vi "Simple Reader.vi"(8 "error in (no error)":errorcluster, 11 "ITC-503 Driver in":refnum<class "ITC-503 Driver.lvclass">) -> (0 "error out":errorcluster, 2 "Signals":dbl[](array[numeric]), 3 "ITC-503 Driver out":refnum<class "ITC-503 Driver.lvclass">)   [LabVIEW 2025, in "ITC-503 Driver.lvclass"]
uses:
  ITC-503 Driver.lvclass
  VISA Instrument/VISA Instrument.lvclass/VISA Instrument.ctl
  VISA Instrument/Read VISA resource.vi
  VISA Instrument/Write VISA resource.vi
  Temperature Controller Driver/Read T controller configuration.vi
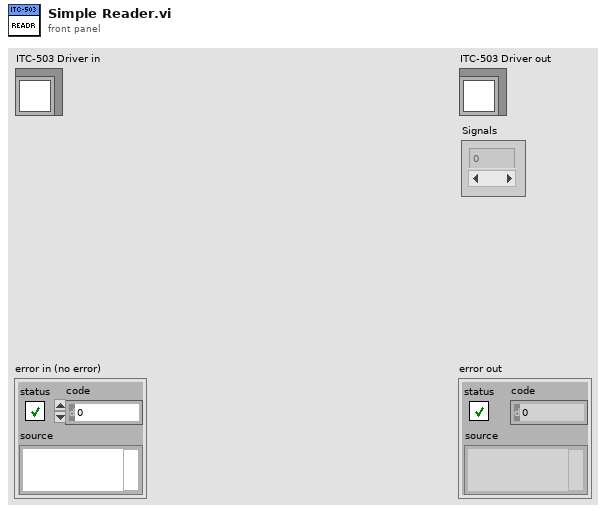
[diagram p1: front panel]
types:
  T1 = typedef "T controller configuration.ctl" = cluster{"Record Channels":string[], "Record raw signal":bool, "Set point":dbl, "Record heater":bool, "Ramp rate":dbl, "P":dbl, "I":dbl, "D":dbl, "Control":T2, "P manual":dbl, "Output #":i32}
  T2 = typedef "Control Mode.ctl" = enum16{"Off", "PID", "Ramp", "Manual", "Table"}
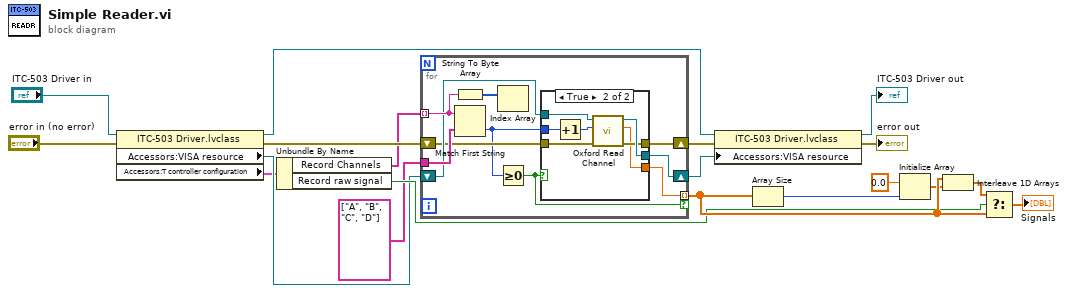
[diagram p0: block diagram]
diagram:
  n1 = property class="ITC-503 Driver.lvclass"(reference="ITC-503 Driver in", error in="error in (no error)") -> (reference out=w11:refnum<class "ITC-503 Driver.lvclass">, error out=w10:errorcluster, "Accessors:VISA resource"=w9:refnum<visa-resource-name>, "Accessors:T controller configuration"=w8:T1)
  n2 = Unbundle By Name(w8) -> ("Record Channels"=w7:string[], "Record raw signal"=w16:bool)
  n3 = for {
    tunnel: w7 -> [w27] mode=indexing
    tunnel: [w23] -> w19 mode=indexing if=w21
    shift-right: [w24] -> w13
    shift-left: w10 -> [w22]
    shift-right: [w25] -> w12
    shift-left: w9 -> [w26]
    tunnel: string[] ["A", "B", "C", "D"] ("Array - String") -> [w28]
    n4 = String To Byte Array(string=w27) -> (unsigned byte array=w29:u8[])
    n5 = Match First String(2:w28, 3:w27) -> (0:w20:i32)  [unwired: 1 out]
    n6 = Index Array(array=w29) -> ()  [unwired: 1 in, 1 out]
    n7 = Greater Or Equal To 0?(x=w20) -> (x >= 0?=w21:bool)
    n8 = case shown="True" w21 {
      tunnel: w26 -> [w31 w38]
      tunnel: [w31 w37] -> w25
      tunnel: [w30 w36] -> w24
      tunnel: [_ w35] -> w23
      tunnel: w22 -> [w30 w34]
      tunnel: w20 -> [_ w33]
      frame False {
      }
      frame True {
        n9 = Increment(x=w33) -> (x+1=w32:i32)
        n10 = call "Oxford Read Channel.vi"("error in (no error)"=w34, "Channel #"=w32, "VISA resource name"=w38) -> ("error out"=w36:errorcluster, "Data"=w35:dbl, "VISA resource name out"=w37:refnum<visa-resource-name>)  [unwired: 5 in, 1 out]
      }
    }
  }
  n11 = property class="ITC-503 Driver.lvclass"(reference=w11, error in=w13, "Accessors:VISA resource"=w12) -> (reference out=→"ITC-503 Driver out":refnum<class "ITC-503 Driver.lvclass">, error out=→"error out":errorcluster)
  n12 = Array Size(array=w19) -> (size(s)=w14:i32)
  n13 = Initialize Array(0.0 ("element"), w14) -> (w17:dbl[])
  n14 = Interleave 1D Arrays(w19, w17) -> (w18:dbl[])
  n15 = Select(t=w18, s=w16, f=w19) -> (s? t:f=→"Signals":dbl[])
